vi "COD浓度全局变量.vi"() -> ()   [LabVIEW 2016, in "斯坦道CODMn.lvlib"]
uses:
  <vilib>/Plasmionique/MB Master/MB_Master/MB_Master.lvclass
panel:
  in  "MB session in":refnum<class "MB_Master.lvclass">
  in  "标准液浓度":dbl
  in  "COD浓度（mg/L)":dbl
  # "标准液浓度（mg/L）："
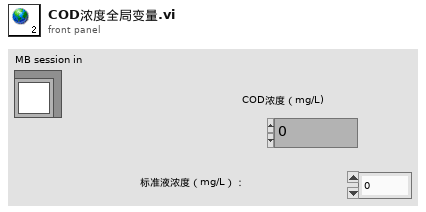
[diagram p1: front panel]
diagram:
